vi "Multi-sweep channel.vi"(7 "Time interval":u32=10 min=10 max=20000 step=5 format="%.0f ms", 8 "Error In":errorcluster, 9 "Index":i32, 10 "Multi-sweep settings":T1 {"Vstep" min=0.0125 max=204.8 step=0.0125 format="%#_g V"; "Vstop" min=0 max=204.8 step=0.0125 format="%#_g V"; "Vstart" min=0 max=204.8 step=0.0125 format="%#_g V"; "Channel to sweep" max=31 step=1}, 11 "Arduino Port":refnum<visa-resource-name>) -> (0 "Error Out":errorcluster, 3 "Arduino Port out":refnum<visa-resource-name>)   [LabVIEW 2016]
uses:
  Typedef/AD5535 - Multi sweep settings.ctl
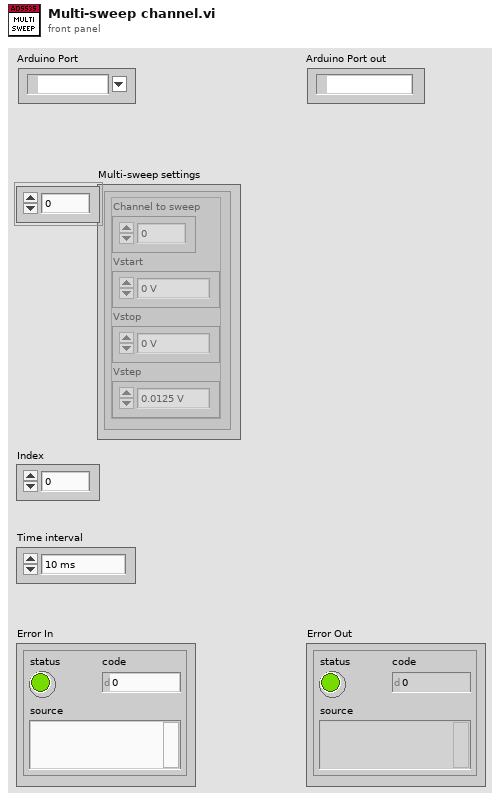
[diagram p1: front panel]
types:
  T1 = typedef "AD5535 - Multi sweep settings.ctl" = cluster{"Channel to sweep":u8, "Vstart":sgl, "Vstop":sgl, "Vstep":sgl}[]
  T2 = cluster{"Channel to sweep":u8, "Vstart":sgl, "Vstop":sgl, "Vstep":sgl}
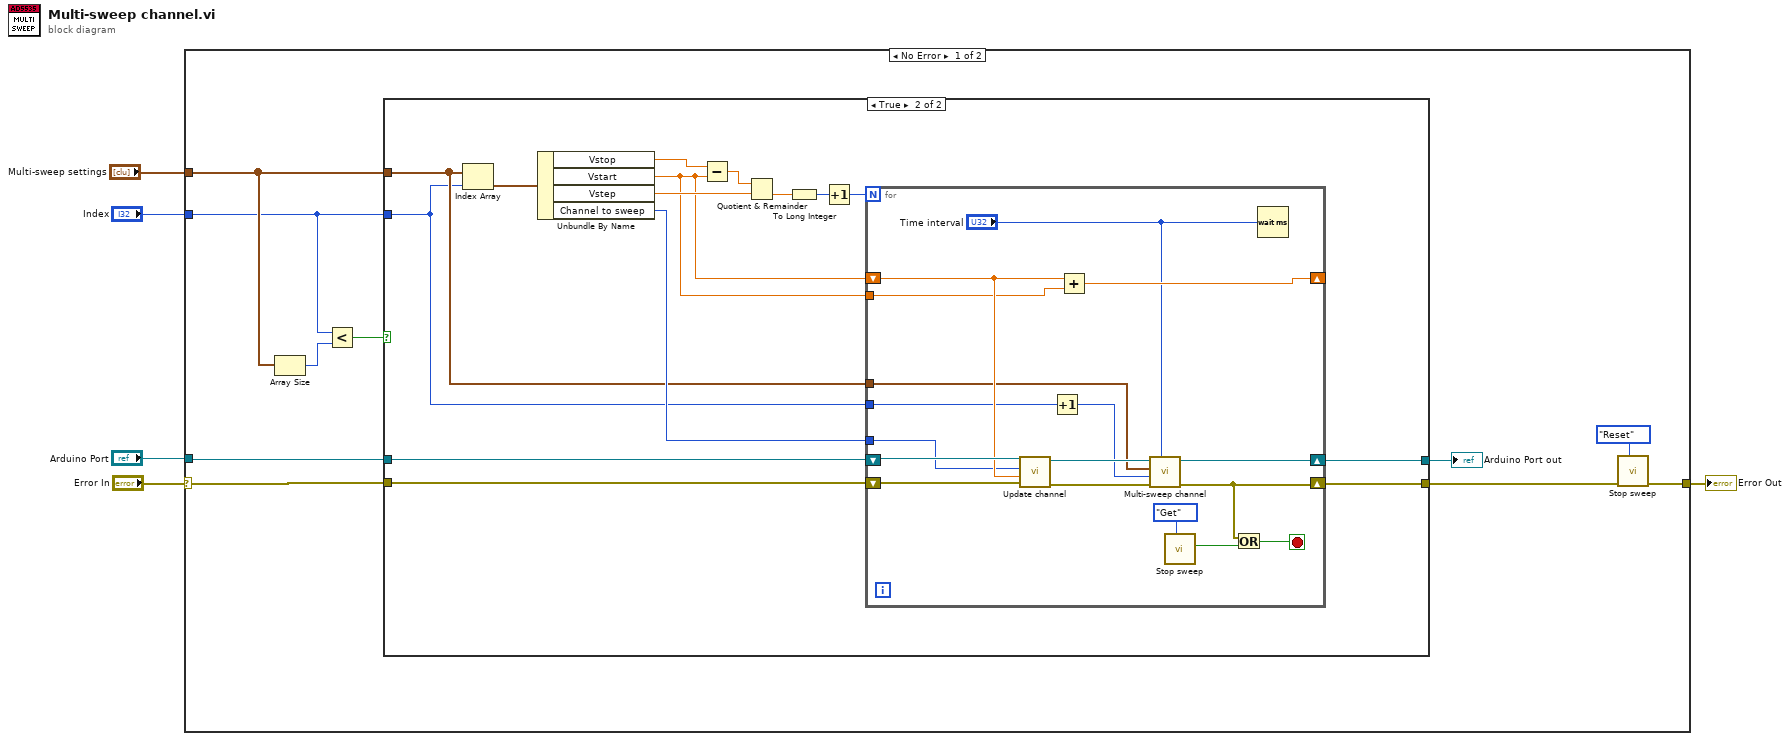
[diagram p0: block diagram]
diagram:
  n1 = case shown="No Error" "Error In" {
    selector: "Error In" -> [w13 w50]
    tunnel: "Arduino Port" -> [w14 _]
    tunnel: "Multi-sweep settings" -> [w12 _]
    tunnel: [w6 w50] -> w4
    tunnel: "Index" -> [w11 _]
    frame No Error {
      n2 = Array Size(array=w12) -> (size(s)=w10:i32)
      n3 = Less?(x=w11, y=w10) -> (x < y?=w9:bool)
      n4 = case shown="True" w9 {
        tunnel: [w16 w28] -> w7
        tunnel: [w17 w27] -> w15
        tunnel: w14 -> [w17 w26]
        tunnel: w13 -> [w16 w25]
        tunnel: w12 -> [_ w19]
        tunnel: w11 -> [_ w18]
        frame False {
        }
        frame True {
          n5 = Index Array(array=w19, index=w18) -> (element=w24:T2)
          n6 = Unbundle By Name(w24) -> ("Vstop"=w23:sgl, "Vstart"=w20:sgl, "Vstep"=w22:sgl, "Channel to sweep"=w21:u8)
          n7 = Subtract(x=w23, y=w20) -> (x-y=w32:sgl)
          n8 = Quotient & Remainder(x=w32, y=w22) -> (floor(x/y)=w31:sgl)  [unwired: 1 out]
          n9 = To Long Integer(number=w31) -> (32bit integer=w30:i32)
          n10 = Increment(x=w30) -> (x+1=w29:i32)
          n11 = for {
            N: w29 -> [_]
            shift-right: [w35] -> w28
            shift-left: w25 -> [w48]
            shift-right: [w42] -> w27
            shift-left: w26 -> [w49]
            shift-right: [w46] -> _
            shift-left: w20 -> [w47]
            tunnel: w21 -> [w45]
            tunnel: w20 -> [w44]
            tunnel: w19 -> [w40]
            tunnel: w18 -> [w39]
            stop <- w34 stop-if-true
            n12 = call "Update channel.vi"("Error In"=w48, "Value"=w47, "Channel"=w45, "Arduino Port"=w49) -> ("Error Out"=w41:errorcluster, "Arduino Port out"=w43:refnum<visa-resource-name>)  [unwired: 6 in]
            n13 = Increment(x=w39) -> (x+1=w38:i32)
            n14 = Add(x=w47, y=w44) -> (x+y=w46:sgl)
            n15 = call "Multi-sweep channel.vi"("Time interval"="Time interval", "Error In"=w41, "Index"=w38, "Multi-sweep settings"=w40, "Arduino Port"=w43) -> ("Error Out"=w35:errorcluster, "Arduino Port out"=w42:refnum<visa-resource-name>)  [unwired: 5 in]
            n16 = call "Stop sweep.vi"("Status"=enum16{"Set", "Get", "Reset"}."Get") -> ("Exit?"=w36:bool)  [unwired: 9 in, 1 out]
            n17 = Or(x=w35, y=w36) -> (x .or. y?=w34:bool)
            n18 = Wait (ms)(milliseconds to wait="Time interval") -> ()  [unwired: 1 out]
          }
        }
      }
      "Arduino Port out" <- w15
      n19 = call "Stop sweep.vi"("Status"=enum16{"Set", "Get", "Reset"}."Reset", "Error In"=w7) -> ("Error Out"=w6:errorcluster)  [unwired: 8 in, 1 out]
    }
    frame Error {
    }
  }
  "Error Out" <- w4
